vi "Delete empty element from end.vi"(11 "Columnname_Alais":string[](array[string])) -> (3 "reversed array":string[](array[string]))   [LabVIEW 2017, in "SQLite.lvclass"]
uses:
  SQLite.lvclass
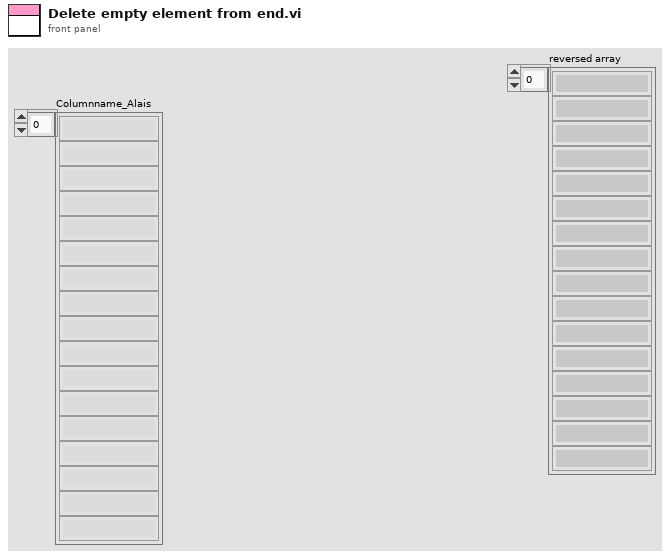
[diagram p1: front panel]
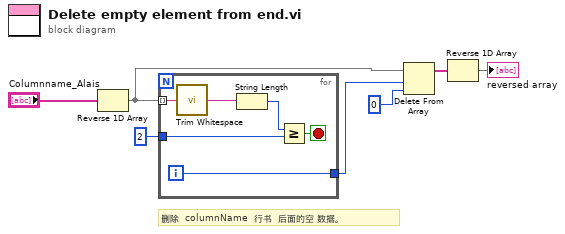
[diagram p0: block diagram]
diagram:
  # "删除  columnName  行书  后面的空 数据。"
  n1 = Reverse 1D Array(array="Columnname_Alais") -> (reversed array=w1:string[])
  n2 = for {
    tunnel: w1 -> [w13] mode=indexing
    tunnel: 2 ("y") -> [w11]
    tunnel: [w9] -> w5
    i -> [w9]
    stop <- w10 stop-if-true
    n3 = call <vilib>:"Trim Whitespace.vi"("string"=w13) -> ("trimmed string"=w8:string)  [unwired: 1 in]
    n4 = String Length(string=w8) -> (length=w12:i32)
    n5 = Greater Or Equal?(x=w12, y=w11) -> (x >= y?=w10:bool)
  }
  n6 = Delete From Array(array=w1, length=w5, index=0) -> (array with subset deleted=w3:string[])  [unwired: 1 out]
  n7 = Reverse 1D Array(array=w3) -> (reversed array=→"reversed array":string[])
